vi "TimeInfoCLOSE.vi"(7 "error in (no error)":errorcluster, 9 "Minor Time":u32, 10 "Major Time":u32) -> (1 "Close":cluster{"Time":string, "Error":string})   [LabVIEW 2015]
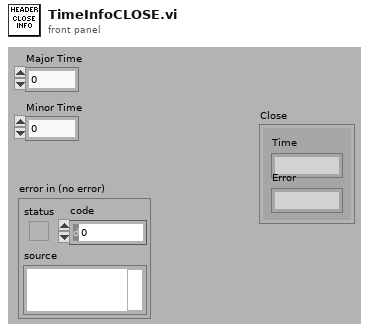
[diagram p1: front panel]
types:
  T1 = cluster{"  Close Time":string, "Close Error":string}
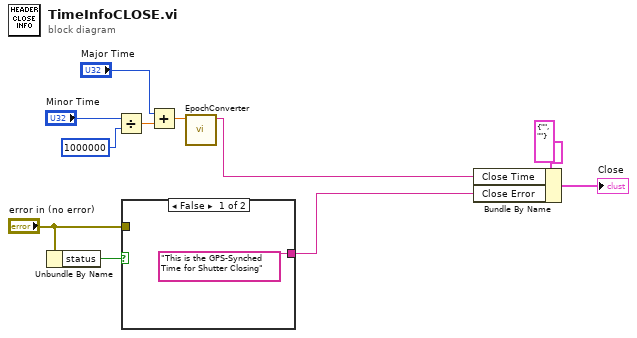
[diagram p0: block diagram]
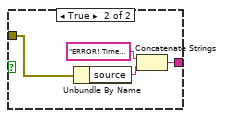
[diagram p2: hidden frame]
diagram:
  n1 = Unbundle By Name("error in (no error)") -> ("status"=w11:bool)
  n2 = Divide(x="Minor Time", y=1000000) -> (x/y=w3:dbl)
  n3 = case shown="False" w11 {
    tunnel: "error in (no error)" -> [_ w16]
    tunnel: ["This is the GPS-Synched Time for Shutter Closing" w13] -> w8
    frame False {
    }
    frame True {
      n4 = Unbundle By Name(w16) -> ("source"=w14:string)
      n5 = Concatenate Strings("ERROR! Time may be Invalid.  Source: ", w14) -> (w13:string)
    }
  }
  n6 = Add(x="Major Time", y=w3) -> (x+y=w1:dbl)
  n7 = call "EpochConverter.vi"("Epoch time"=w1) -> ("String"=w6:string)  [unwired: 9 in, 1 out]
  n8 = Bundle By Name(cluster=T1 {"  Close Time"="", "Close Error"=""}, "Close Time"=w6, "Close Error"=w8) -> (→"Close":T1)
